vi "SelectFile.vi"(4 "Button Label":string caption="button label", 6 "Prompt":string="Select File", 8 "Error In":errorcluster, 9 "File Description":string="All Files", 10 "File Extension (.*)":string=".*", 11 "Start Path":path) -> (0 "Error Out":errorcluster, 2 "Cancelled?":bool caption="cancelled", 3 "Selected File Path":path)   [LabVIEW 2013, in "LV-Utilities.lvlib"]
uses:
  LV-Utilities.lvlib
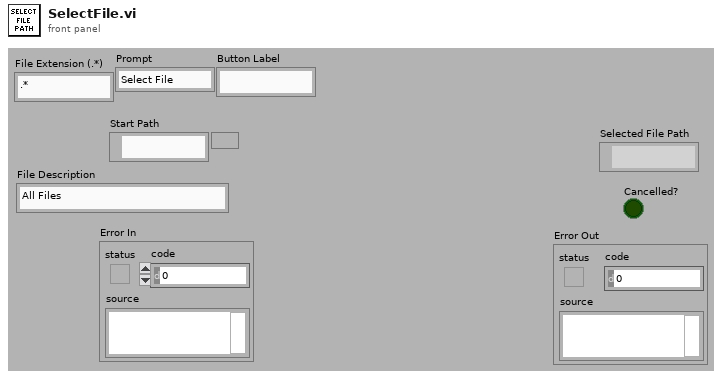
[diagram p1: front panel]
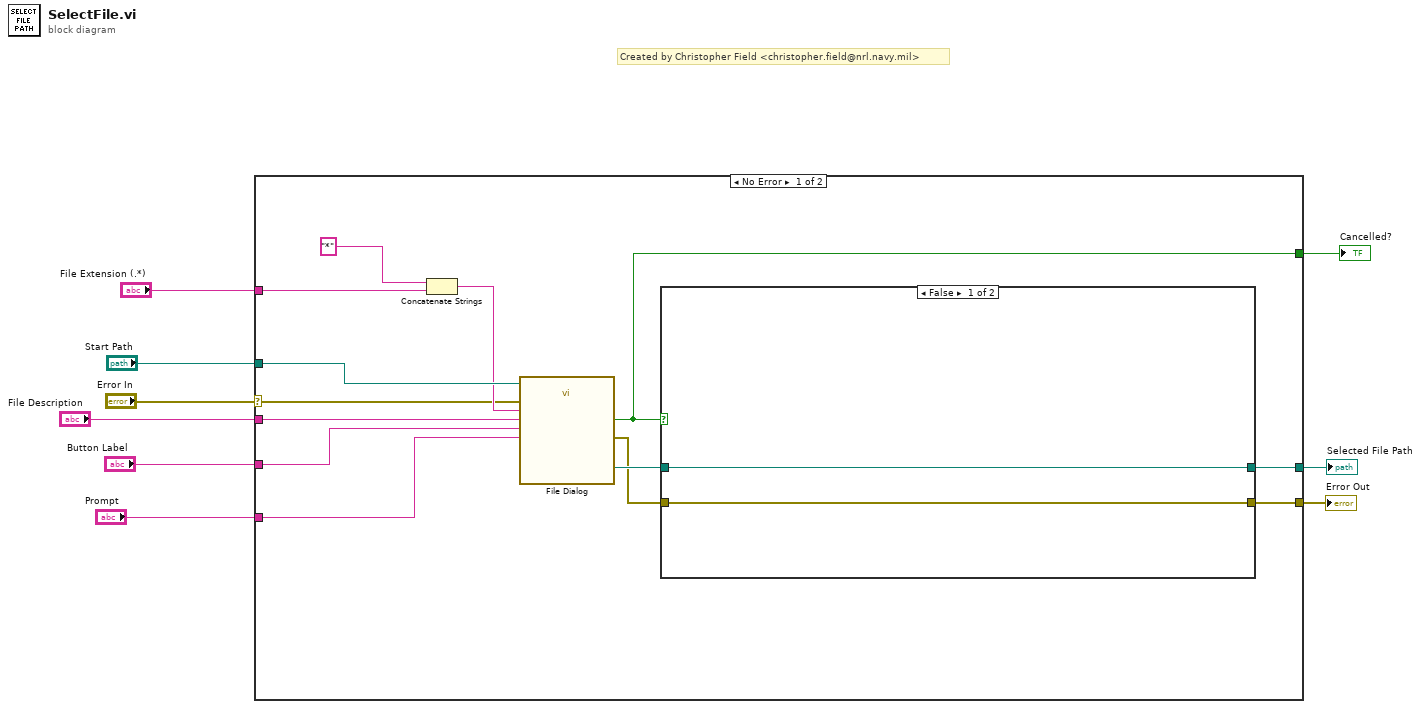
[diagram p0: block diagram]
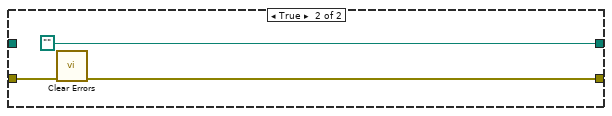
[diagram p2: hidden frame]
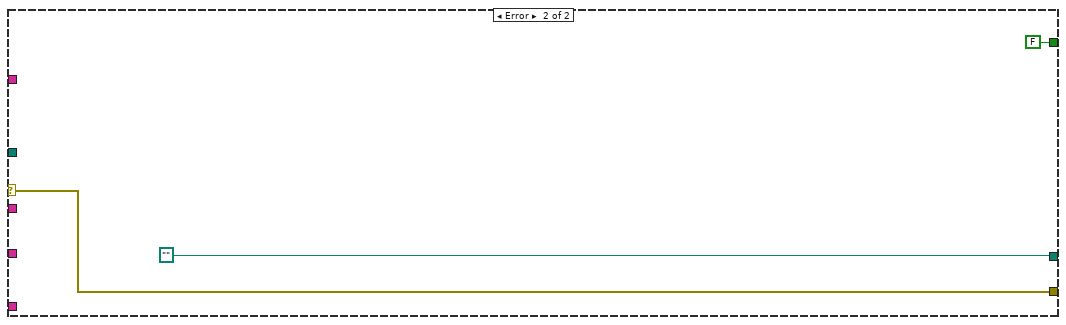
[diagram p3: hidden frame]
diagram:
  # "Created by Christopher Field <christopher.field@nrl.navy.mil>"
  n1 = case shown="No Error" "Error In" {
    selector: "Error In" -> [w12 w29]
    tunnel: "Start Path" -> [w22 _]
    tunnel: "File Description" -> [w21 _]
    tunnel: [w20 FALSE ("cancelled")] -> w7
    tunnel: [w17 w29] -> w6
    tunnel: [w16 path ""] -> w5
    tunnel: "File Extension (.*)" -> [w14 _]
    tunnel: "Prompt" -> [w11 _]
    tunnel: "Button Label" -> [w10 _]
    frame No Error {
      n2 = Concatenate Strings("*" ("string"), w14) -> (w13:string)
      n3 = call "File Dialog"("start path"=w22, "prompt"=w11, "button label"=w10, "error in"=w12, "pattern (all files)"=w13, "pattern label"=w21) -> ("selected path"=w19:path, "cancelled"=w20:bool, "error out"=w18:errorcluster)  [unwired: 6 in, 1 out]
      n4 = case shown="False" w20 {
        tunnel: w19 -> [w23 _]
        tunnel: w18 -> [w24 w27]
        tunnel: [w24 w26] -> w17
        tunnel: [w23 path ""] -> w16
        frame False {
        }
        frame True {
          n5 = call <vilib>:"Clear Errors.vi"("error in (no error)"=w27) -> ("error out"=w26:errorcluster)  [unwired: 6 in]
        }
      }
    }
    frame Error {
    }
  }
  "Cancelled?" <- w7
  "Error Out" <- w6
  "Selected File Path" <- w5
